vi "Hex to Dec.vi"(11 "String":string) -> (3 "Array":bool[](array[boolean]))   [LabVIEW 2020, in "Cypress.lvclass"]
uses:
  Cypress.lvclass
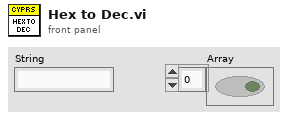
[diagram p1: front panel]
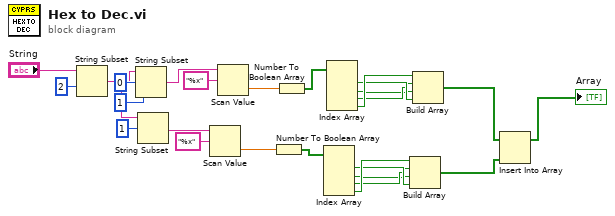
[diagram p0: block diagram]
diagram:
  n1 = String Subset(string="String", offset (0)=2) -> (substring=w2:string)  [unwired: 1 in]
  n2 = String Subset(string=w2, offset (0)=0, length (rest)=1 ("length (rest)")) -> (substring=w9:string)
  n3 = String Subset(string=w2, offset (0)=1) -> (substring=w6:string)  [unwired: 1 in]
  n4 = Scan Value(string=w6, format string="%x") -> (value=w11:dbl)  [unwired: 1 in, 1 out]
  n5 = Scan Value(string=w9, format string="%x") -> (value=w10:dbl)  [unwired: 1 in, 1 out]
  n6 = Number To Boolean Array(number=w11) -> (Boolean array=w22:bool[])
  n7 = Number To Boolean Array(number=w10) -> (Boolean array=w17:bool[])
  n8 = Index Array(array=w22) -> (element #1=w20:bool, element #2=w18:bool, element #3=w19:bool, element #4=w21:bool)  [unwired: 4 in]
  n9 = Index Array(array=w17) -> (element #1=w15:bool, element #2=w13:bool, element #3=w14:bool, element #4=w16:bool)  [unwired: 4 in]
  n10 = Build Array(w21, w19, w18, w20) -> (w24:bool[])
  n11 = Build Array(w16, w14, w13, w15) -> (w23:bool[])
  n12 = Insert Into Array(array=w23, new element=w24) -> (→"Array":bool[])  [unwired: 1 in]
